vi "Show_Error.vi"(8 "error in (no error)":errorcluster, 10 "Error":i32) -> (0 "error out":errorcluster)   [LabVIEW 2017]
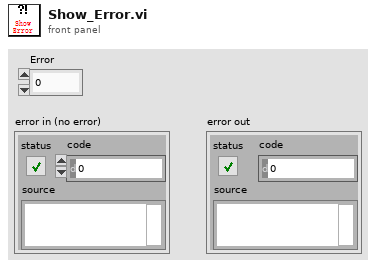
[diagram p1: front panel]
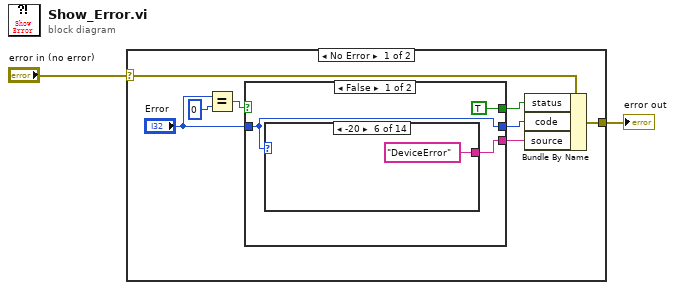
[diagram p0: block diagram]
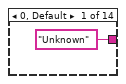
[diagram p2: hidden frame]
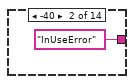
[diagram p3: hidden frame]
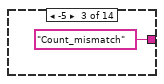
[diagram p4: hidden frame]
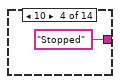
[diagram p5: hidden frame]
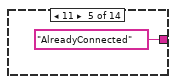
[diagram p6: hidden frame]
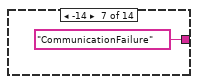
[diagram p7: hidden frame]
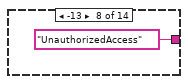
[diagram p8: hidden frame]
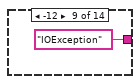
[diagram p9: hidden frame]
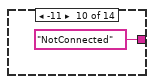
[diagram p10: hidden frame]
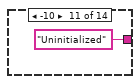
[diagram p11: hidden frame]
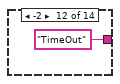
[diagram p12: hidden frame]
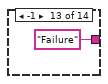
[diagram p13: hidden frame]
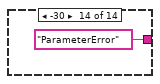
[diagram p14: hidden frame]
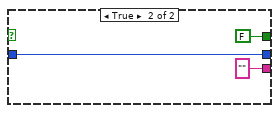
[diagram p15: hidden frame]
diagram:
  n1 = case shown="No Error" "error in (no error)" {
    selector: "error in (no error)" -> [w7 w31]
    tunnel: [w5 w31] -> w1
    frame No Error {
      n2 = Equal?(x="Error", y=0) -> (x = y?=w10:bool)
      n3 = case shown="False" w10 {
        tunnel: "Error" -> [w12 w29]
        tunnel: [w13 ""] -> w8
        tunnel: [w12 w29] -> w6
        tunnel: [TRUE FALSE] -> w3
        frame False {
          n4 = case shown="-20" w12 {
            tunnel: ["Unknown" "InUseError" "Count_mismatch" "Stopped" "AlreadyConnected" "DeviceError" "CommunicationFailure" "UnauthorizedAccess" "IOException" "NotConnected" "Uninitialized" "TimeOut" "Failure" "ParameterError"] -> w13
            frame 0, Default {
            }
            frame -40 {
            }
            frame -5 {
            }
            frame 10 {
            }
            frame 11 {
            }
            frame -20 {
            }
            frame -14 {
            }
            frame -13 {
            }
            frame -12 {
            }
            frame -11 {
            }
            frame -10 {
            }
            frame -2 {
            }
            frame -1 {
            }
            frame -30 {
            }
          }
        }
        frame True {
        }
      }
      n5 = Bundle By Name(cluster=w7, "status"=w3, "code"=w6, "source"=w8) -> (w5:errorcluster)
    }
    frame Error {
    }
  }
  "error out" <- w1
